vi "Write temperatures.vi"(8 "error in (no error)":errorcluster, 10 "temperatures":T1, 11 "Nicholas Data in":refnum<class "SOAP Data.lvclass">) -> (0 "error out":errorcluster, 3 "Nicholas Data out":refnum<class "SOAP Data.lvclass">)   [LabVIEW 2017, in "Controller.lvlib" / "SOAP Data.lvclass"]
uses:
  SOAP Data.lvclass
  SOAP Data.lvclass/SOAP Data.ctl
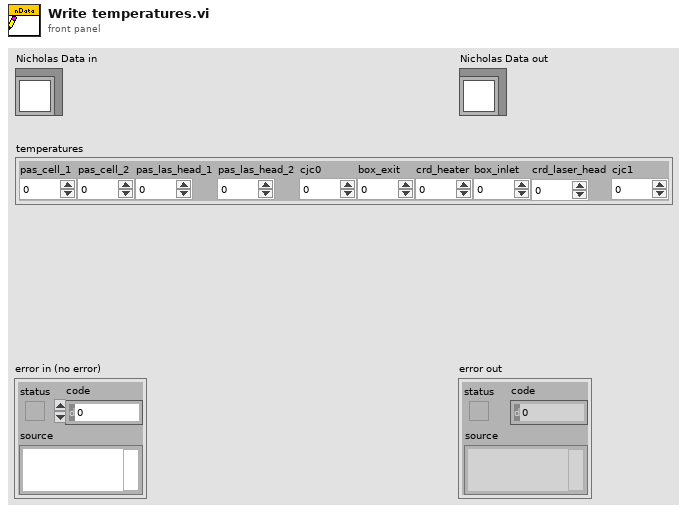
[diagram p1: front panel]
types:
  T1 = cluster{"pas_cell_1":sgl, "pas_cell_2":sgl, "pas_las_head_1":sgl, "pas_las_head_2":sgl, "cjc0":sgl, "box_exit":sgl, "crd_heater":sgl, "box_inlet":sgl, "crd_laser_head":sgl, "cjc1":sgl}
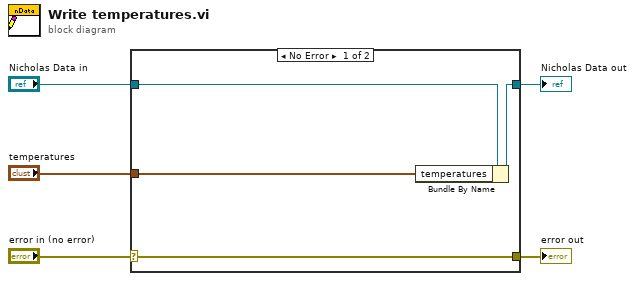
[diagram p0: block diagram]
diagram:
  n1 = case shown="No Error" "error in (no error)" {
    selector: "error in (no error)" -> [w9 w10]
    tunnel: [w9 w10] -> w4
    tunnel: [w7 w11] -> w2
    tunnel: "Nicholas Data in" -> [w8 w11]
    tunnel: "temperatures" -> [w6 _]
    frame No Error {
      n2 = Bundle By Name(cluster=w8, "temperatures"=w6) -> (w7:refnum<class "SOAP Data.lvclass">)
    }
    frame Error {
    }
  }
  "error out" <- w4
  "Nicholas Data out" <- w2
